vi "Change Laser Output.vi"(8 "error in":errorcluster, 11 "cPAS in":refnum<class "cPAS.lvclass">) -> (0 "error out":errorcluster, 3 "cPAS out":refnum<class "cPAS.lvclass">)   [LabVIEW 2015, in "cPAS.lvclass"]
uses:
  cPAS.lvclass
  cPAS.lvclass/cPAS.ctl
  Reusable/Instrument/Instrument.lvclass
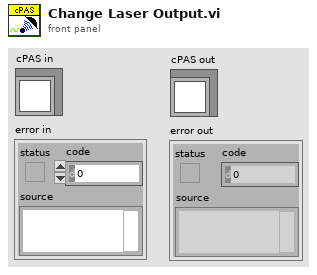
[diagram p1: front panel]
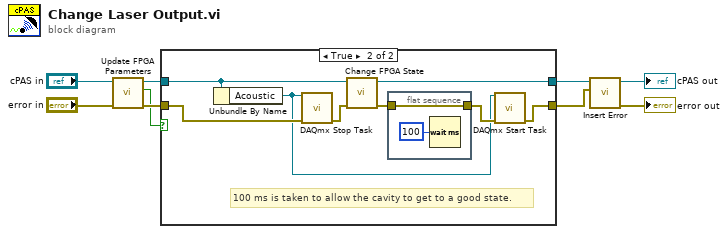
[diagram p0: block diagram]
diagram:
  n1 = call "Update FPGA Parameters.vi"("error in"="error in", "cPAS in"="cPAS in") -> ("error out"=w3:errorcluster, "Update FPGA?"=w2:bool, "cPAS out"=w4:refnum<class "cPAS.lvclass">)  [unwired: 7 in]
  n2 = case shown="True" w2 {
    tunnel: [w11 w17] -> w8
    tunnel: [w10 w18] -> w6
    tunnel: w4 -> [w11 w14]
    tunnel: w3 -> [w10 w15]
    frame False {
    }
    frame True {
      # "100 ms is taken to allow the cavity to get to a good state."
      n3 = Unbundle By Name(w14) -> ("Acoustic"=w12:refnum<k21>)
      n4 = call <vilib>:"DAQmx Stop Task.vi"("task/channels in"=w12, "error in"=w15) -> ("error out"=w13:errorcluster)  [unwired: 12 in, 1 out]
      n5 = call "Change FPGA State.vi"("error in"=w13, "cPAS in"=w14) -> ("error out"=w19:errorcluster, "cPAS out"=w17:refnum<class "cPAS.lvclass">)  [unwired: 8 in]
      n6 = flat-sequence {
        tunnel: [w20] -> w16
        tunnel: w19 -> [w20]
        frame #0 {
          n7 = Wait (ms)(milliseconds to wait=u32 100) -> ()  [unwired: 1 out]
        }
      }
      n8 = call <vilib>:"DAQmx Start Task.vi"("task/channels in"=w12, "error in"=w16) -> ("error out"=w18:errorcluster)  [unwired: 12 in, 1 out]
    }
  }
  n9 = call "Insert Error.vi"("err"=w6, "Instrument in"=w8) -> ("error out"=→"error out":errorcluster, "Instrument out"=→"cPAS out":refnum<class "cPAS.lvclass">)  [unwired: 7 in, 1 out]
